vi "editDialog.vi"(0 "reference":refnum<class "StateTransitionEdge.lvclass">, 5 "error in (no error)":errorcluster) -> (14 "reference out":refnum<class "StateTransitionEdge.lvclass">, 15 "cancel":bool, 19 "error out":errorcluster)   [LabVIEW 2012, in "StateTransitionEdge.lvclass"]
doc: "Edit Dialog"
uses:
  <resource>/Framework/Providers/Open_GDS/UML/StateTransitionEdge_class/StateTransitionEdge.lvclass
  <resource>/Framework/Providers/Open_GDS/UML/BentStyle_class/BentStyleType.ctl
  <resource>/Framework/Providers/Open_GDS/UML/ContextHelp/ContextHelp_HelpTexts.ctl
  <resource>/Framework/Providers/Open_GDS/UML/BentStyle_class/BentStyle.lvclass
panel:
  in  "Bent Style":T1
  in  "Help":bool
  in  "Event":string
  in  "Cancel Button":bool
  in  "OK Button":bool
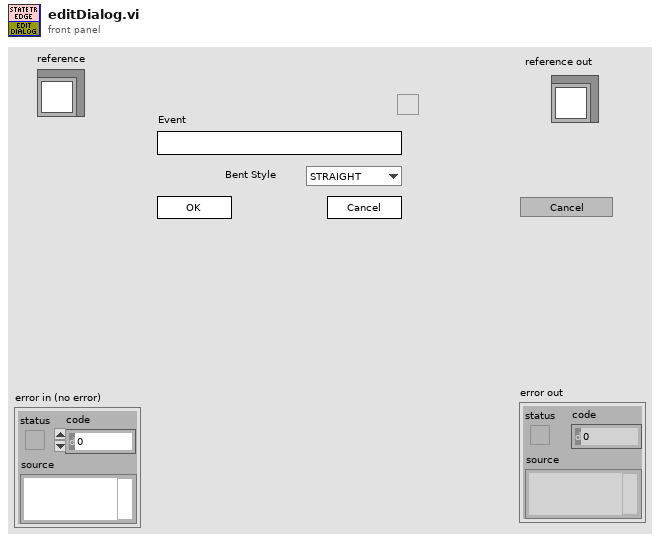
[diagram p1: front panel]
types:
  T1 = typedef "BentStyle.lvclass/BentStyleType.ctl" = enum16{"STRAIGHT", "HV", "VH", "HVH", "VHV", "ARC"}
  T2 = typedef "ContextHelp_HelpTexts.ctl" = enum16{"None(Hide)", "Default", "Help", "Welcome", "GettingStarted", "ClassDiagram_Help", "SequenceDiagram_Help", "UseCaseDiagram_Help", "BSelect", "BClass", "BInterface", "BPackage", "BNote", "BDependency", "BInheritance", "BInterfaceImplementation", "BAssociation", "BAggregation", "BCompAggregation", "BNoteConnector", "BObject", "BActionBar", "BCall", "BSystem", "BActor", "BUseCase", "BGeneralization", "BIncludes", "BExtends", "BUseCaseDiagramAssociation", "ClassRelationshipEdge editDialog_Bent Style", "ClassRelationshipEdge editDialog_RelationType", "ClassRelationshipEdge editDialog_Reverse association", "ClassRelationshipEdge editDialog_Start label", "ClassRelationshipEdge editDialog_Middle label", "ClassRelationshipEdge editDialog_End label", "UMLEditor reversedEngineering_Pathes", "ReversedEngineering StateReverseDialog_Help", "ReversedEngineering StateQueuedSettings_Help", "UMLEditor reversedEngineering_AddTopVIs", "UMLEditor reversedEngineering_AddClasses", "UMLEditor reversedEngineering_AddDirs", "UMLEditor reversedEngineering_Recursively", "UMLEditor reversedEngineering_Remove", "UMLEditor reversedEngineering_ClearList", "UMLEditor reversedEngineering_HideSubAss", "UMLEditor reversedEngineering_CreateTypes", "UMLEditor reversedEngineering_OnlyInheritance", "UMLEditor reversedEngineering_CreateApplication", "UMLEditor reversedEngineering_OK", "UMLEditor reversedEngineering_Cancel", "UMLEditor reversedEngineering_Help", "UMLEditor createWizardScriptFile_ScriptfilePath", "UMLEditor createWizardScriptFile_ClassPath", "UMLEditor createWizardScriptFile_Use", "UMLEditor createWizardScriptFile_PrivateDirName", "UMLEditor createWizardScriptFile_DirAppend", "UMLEditor createWizardScriptFile_Separator Character", "UMLEditor createWizardScriptFile_OK", "UMLEditor createWizardScriptFile_Cancel", "UMLEditor createWizardScriptFile_Help", "ClassNode editDialog_Class Name", "InterfaceNode editDialog_Class Name", "ClassNode editDialog_Attribute", "ClassNode editDialog_Methods", "InterfaceNode editDialog_Methods", "ClassNode editDialog_connection", "InterfaceNode editDialog_connection", "ClassNode editDialog_StereoType", "ClassNode editDialog_ShowAttrib", "ClassNode editDialog_ShowMethods", "ClassNode editDialog_ClassPath", "ClassNode editDialog_AddAttribute", "ClassNode editDialog_AddMethod", "InterfaceNode editDialog_AddMethod", "ClassNode AttributeGuide_AttributeName", "ClassNode AttributeGuide_Array?", "ClassNode AttributeGuide_Data Type", "ClassNode AttributeGuide_RefName", "ClassNode AttributeGuide_Preview", "ClassNode AttributeGuide_OK", "ClassNode AttributeGuide_Cancel", "ClassNode MethodGuide_Visibility", "ClassNode MethodGuide_Method Name", "ClassNode MethodGuide_Preview", "ClassNode MethodGuide_OK", "ClassNode MethodGuide_Cancel", "CallNode EditCallProperties_AllButtons", "ObjectNode EditObjectlProperties_AllButtons", "ActorNode EditActorProperties_AllButtons", "UseCaseRelationshipNode EditUseCaselProperties_AllButtons", "UseCaseNode EditUseCaselProperties_AllButtons", "SystemNode EditSystemProperties_AllButtons", "ReversedEngineering UpdateAttributes_AllButtons", "StateNode editDialog_AllButtons", "StateTransition editDialog_AllButtons", "ArrangeNodes Main_Picture", "ArrangeNodes Main_Zoom", "ArrangeNodes Main_Auto Zoom", "ArrangeNodes Main_shorten", "ArrangeNodes Main_Min Length", "ArrangeNodes Main_Max Length", "ArrangeNodes Main_increase", "ArrangeNodes Main_decrease", "ArrangeNodes Main_Shake", "ArrangeNodes Main", "BState", "BInitialState", "BFinalState", "BStateTransition", "StateDiagram_Help", "StateDiagram_PropertiesAllButtons", "ReversedEngineering StateReverseDialog_ClearStates", "ReversedEngineering StateReverseDialog_UseQueuedStateMachines", "ReversedEngineering StateReverseDialog_QueuedSettings", "ReversedEngineering StateReverseDialog_SearchForVIs", "ReversedEngineering StateReverseDialog_SearchCriteria", "OptionsDialog_ClassBasePath", "OptionsDialog_VIPath", "OptionsDialog_ApplicationPath", "OptionsDialog_WizDir", "OptionsDialog_IniFilePath", "OptionsDialog_DefineColors", "OptionsDialog_Help", "OptionsDialog_CreateTypes", "ClassRelationshipEdge editDialog_SplitWire"}
  T3 = typedef "StateTransitionEdge.lvclass/ObjectAttributes.ctl" = cluster{"Base class":T4, "angle":dbl}
  T4 = typedef "ClassRelationshipEdge.lvclass/ObjectAttributes.ctl" = cluster{"Base class":T5, "bentStyleRef":refnum<class "BentStyle.lvclass">, "startConnectionOffset":cluster{"x":i32, "y":i32}, "endConnectionOffset":cluster{"x":i32, "y":i32}, "MidLineOffset":cluster{"x":i32, "y":i32}, "DepClass":T9}
  T5 = typedef "SegmentedLineEdge.lvclass/ObjectAttributes.ctl" = cluster{"Base class":T6, "lineStyle":refnum<class "LineStyle.lvclass">, "startArrowHead":refnum<class "ArrowHead.lvclass">, "endArrowHead":refnum<class "ArrowHead.lvclass">, "startLabel":string, "midLabel":string, "endLabel":string, "MidLabelOffset":T8, "SplitWire":bool}
  T6 = typedef "GeneralPathEdge.lvclass/ObjectAttributes.ctl" = cluster{"Base class":T7}
  T7 = typedef "AbstractEdge.lvclass/ObjectAttributes.ctl" = cluster{"start":refnum<class "AbstractNode.lvclass">, "end":refnum<class "AbstractNode.lvclass">}
  T8 = typedef "Point Point2D.ctl" = cluster{"x":dbl, "y":dbl}
  T9 = typedef "ReversedEngineering_ViDependencyDetailsType.ctl" = cluster{"ThisVIs/Ctls":path[], "Dependent_VIs/Ctls":path[]}
  T10 = typedef "ContextHelp_ShowType.ctl" = cluster{"Header":string, "Picture":picture, "Text":string}
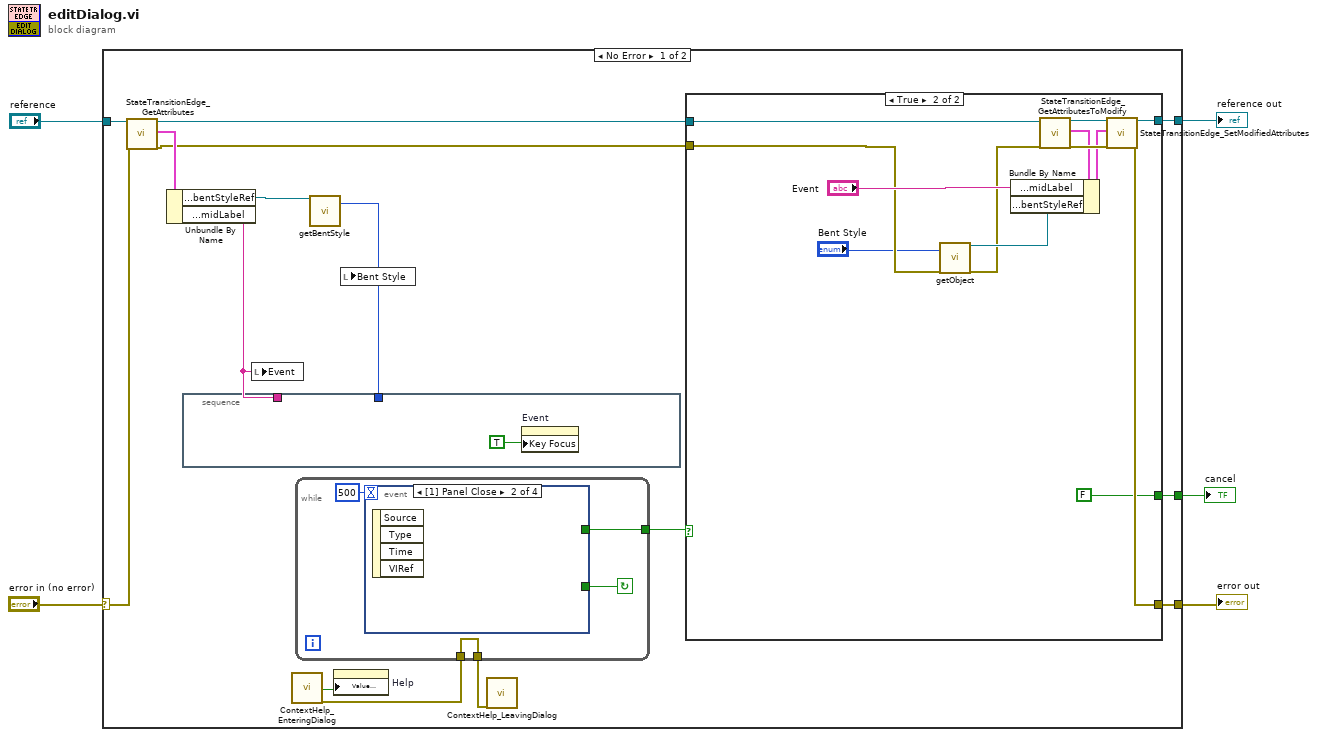
[diagram p0: block diagram]
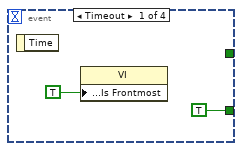
[diagram p2: hidden frame]
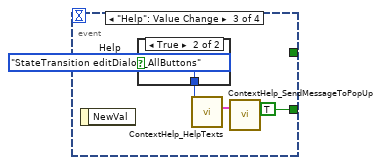
[diagram p3: hidden frame]
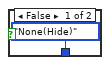
[diagram p4: hidden frame]
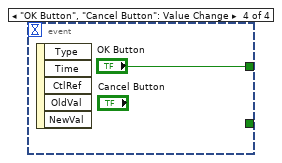
[diagram p5: hidden frame]
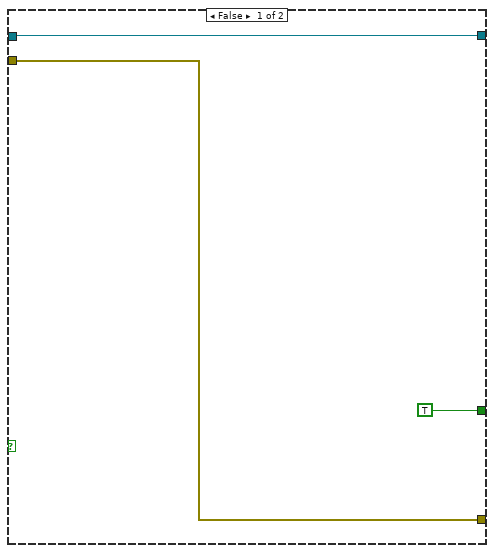
[diagram p6: hidden frame]
diagram:
  n1 = case shown="No Error" "error in (no error)" {
    selector: "error in (no error)" -> [w15 w51]
    tunnel: "reference" -> [w16 w52]
    tunnel: [w20 w51] -> w3
    tunnel: [w19 w52] -> w2
    tunnel: [w12 _] -> w1
    frame No Error {
      n2 = call <resource>:"StateTransitionEdge_GetAttributes.vi"("reference in"=w16, "error in (no error)"=w15) -> ("reference out"=w18:refnum<class "StateTransitionEdge.lvclass">, "Attributes"=w17:T3, "error out"=w11:errorcluster)  [unwired: 15 out]
      n3 = Unbundle By Name(w17) -> ("Base class.bentStyleRef"=w7:refnum<class "BentStyle.lvclass">, "Base class.Base class.midLabel"=w13:string)
      n4 = local write "Event"(w13) -> ()
      n5 = call <resource>:"ContextHelp_EnteringDialog.vi"() -> ("HelpStatus"=w10:bool, "error out"=w8:errorcluster)  [unwired: 3 in, 15 out]
      n6 = while {
        tunnel: [w24] -> w14
        tunnel: [w21] -> w9
        tunnel: w8 -> [w21]
        stop <- w23 continue-if-true
        n7 = event shown="[1] Panel Close" {
          selector: _ -> [_ _ _ _]
          dyn-events: _ -> [_ _ _ _]
          timeout: 500 -> [_ _ _ _]
          tunnel: [_ _ _ "OK Button"] -> w24
          tunnel: [TRUE _ TRUE _] -> w23
          event Timeout {
            n8 = event-data() -> ()  [unwired: 2 out]
            n9 = property class="VI"("Front Panel Window:Is Frontmost"=TRUE) -> ()  [unwired: 2 in, 2 out]
          }
          event Panel Close {
            n10 = event-data() -> ()  [unwired: 5 out]
          }
          event "Help": Value Change {
            n11 = event-data() -> ()  [unwired: 2 out]
            n12 = case shown="True" "Help" {
              tunnel: [ContextHelp_HelpTexts."None(Hide)" ("HelpText") ContextHelp_HelpTexts."StateTransition editDialog_AllButtons" ("HelpText")] -> w29
              frame False {
              }
              frame True {
              }
            }
            n13 = call <resource>:"ContextHelp_HelpTexts.vi"("HelpText (enum or string)"=w29) -> ("HelpOut"=w30:T10)  [unwired: 18 out]
            n14 = call <resource>:"ContextHelp_SendMessageToPopUp.vi"("PopUpMessage"=w30) -> ()  [unwired: 2 in, 17 out]
          }
          event "OK Button", "Cancel Button": Value Change {
            n15 = event-data() -> ()  [unwired: 6 out]
          }
        }
      }
      n16 = call-dynamic "getBentStyle.vi"("reference"=w7) -> ("bentStyle"=w6:T1)  [unwired: 1 in, 17 out]
      n17 = stacked-sequence {
        tunnel: w13 -> [_]
        tunnel: w6 -> [_]
        frame #0 {
          n18 = property on="Event" class="Str"("Key Focus"=TRUE) -> ()  [unwired: 2 in, 2 out]
        }
      }
      n19 = property on="Help" class="Bool (strict)"("Value (Signaling)"=w10) -> ()  [unwired: 2 in, 2 out]
      n20 = local write "Bent Style"(w6) -> ()
      n21 = call <resource>:"ContextHelp_LeavingDialog.vi"("error in (no error)"=w9) -> ()  [unwired: 2 in, 17 out]
      n22 = case shown="True" w14 {
        tunnel: [w34 w48] -> w20
        tunnel: [w36 w47] -> w19
        tunnel: w18 -> [w36 w46]
        tunnel: [TRUE ("Key Focus") FALSE ("Key Focus")] -> w12
        tunnel: w11 -> [w34 w39]
        frame False {
        }
        frame True {
          n23 = call <resource>:"getObject.vi"("bentStyle"="Bent Style", "error in (no error)"=w39) -> ("reference out"=w40:refnum<class "BentStyle.lvclass">, "error out"=w38:errorcluster)  [unwired: 16 out]
          n24 = call <resource>:"StateTransitionEdge_GetAttributesToModify.vi"("reference in"=w46, "error in (no error)"=w38) -> ("reference out"=w49:refnum<class "StateTransitionEdge.lvclass">, "Attributes"=w43:T3, "error out"=w45:errorcluster)  [unwired: 1 in, 14 out]
          n25 = Bundle By Name(cluster=w43, "Base class.Base class.midLabel"="Event", "Base class.bentStyleRef"=w40) -> (w44:T3)
          n26 = call <resource>:"StateTransitionEdge_SetModifiedAttributes.vi"("reference in"=w49, "Attributes"=w44, "error in (no error)"=w45) -> ("reference out"=w47:refnum<class "StateTransitionEdge.lvclass">, "error out"=w48:errorcluster)  [unwired: 3 in, 12 out]
        }
      }
    }
    frame Error {
    }
  }
  "reference out" <- w2
  "error out" <- w3
  "cancel" <- w1
